vi "Log Error.vi"(8 "Error In":errorcluster, 11 "Log Path":path) -> (0 "Error Out":errorcluster={"status"=TRUE, "code"=1, "source"="Set File Position in ConfigTool.lvlib:Logging Event.vi->Main.vi"}, 3 "Log refnum out":refnum<file>)   [LabVIEW 2025, in "Config Tool.lvlib"]
uses:
  Config Tool.lvlib
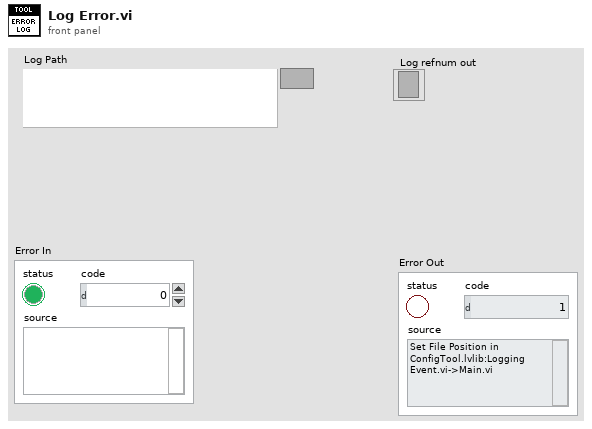
[diagram p1: front panel]
types:
  T1 = enum16{"open", "replace", "create", "open or create", "replace or create", "replace or create with confirmation"}
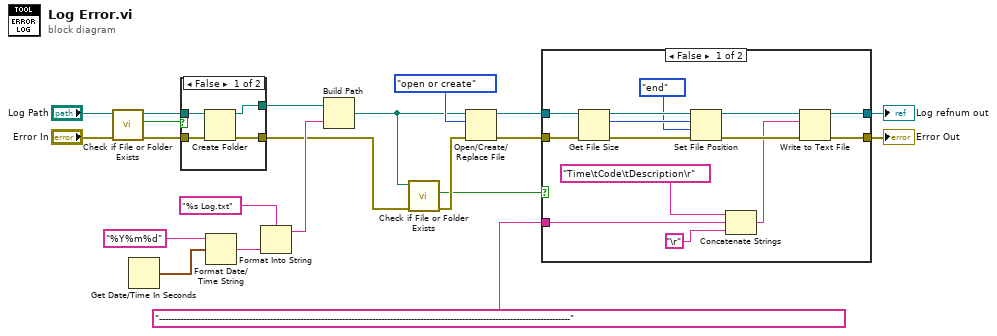
[diagram p0: block diagram]
diagram:
  n1 = call <vilib>:"Check if File or Folder Exists.vi"("error in (no error)"="Error In", "path"="Log Path") -> ("error out"=w7:errorcluster, "file or folder exists?"=w4:bool, "dup path"=w5:path)  [unwired: 7 in]
  n2 = Get Date/Time In Seconds() -> (seconds since 1Jan1904=w9:timestamp)
  n3 = case shown="False" w4 {
    tunnel: w7 -> [w25 w27]
    tunnel: [w24 w27] -> w6
    tunnel: w5 -> [w23 w26]
    tunnel: [w22 w26] -> w3
    frame False {
      n4 = Create Folder(path (use dialog)=w23, error in=w25) -> (created path=w22:path, error out=w24:errorcluster)  [unwired: 1 in, 1 out]
    }
    frame True {
    }
  }
  n5 = Format Date/Time String(time format string (%c)="%Y%m%d", seconds (now)=w9) -> (date/time string=w10:string)  [unwired: 1 in]
  n6 = Format Into String(format string="%s Log.txt" ("name or relative path"), w10) -> (resulting string=w11:string)  [unwired: 2 in, 1 out]
  n7 = Build Path(base path=w3, name or relative path=w11) -> (appended path=w13:path)
  n8 = call <vilib>:"Check if File or Folder Exists.vi"("error in (no error)"=w6, "path"=w13) -> ("error out"=w15:errorcluster, "file or folder exists?"=w14:bool)  [unwired: 7 in, 1 out]
  n9 = Open/Create/Replace File(file path (use dialog)=w13, error in=w15, operation (0:open)=T1."open or create") -> (refnum out=w12:refnum<file>, error out=w8:errorcluster)  [unwired: 3 in, 1 out]
  n10 = case shown="False" w14 {
    tunnel: w8 -> [w41 w42]
    tunnel: [w40 w42] -> w20
    tunnel: w12 -> [w37 w43]
    tunnel: [w39 w43] -> w1
    tunnel: "-----------------------------------------------------------------------------------------------------------------------------------------" -> [w31 _]
    frame False {
      n11 = Get File Size(file=w37, error in=w41) -> (refnum out=w35:refnum<file>, size (in bytes)=w33:i64, 0:w38:errorcluster)
      n12 = Set File Position(offset (in bytes) (0)=w33, refnum=w35, from (0:start)=enum16{"start", "end", "current"}."end", error in=w38) -> (refnum out=w34:refnum<file>, error out=w36:errorcluster)
      n13 = Concatenate Strings("Time\tCode\tDescription\r" ("text"), w31, "\r") -> (w29:string)
      n14 = Write to Text File(file (use dialog)=w34, text=w29, error in=w36) -> (refnum out=w39:refnum<file>, error out=w40:errorcluster)  [unwired: 1 in, 1 out]
    }
    frame True {
    }
  }
  "Error Out" <- w20
  "Log refnum out" <- w1
